vi "MAIN v1.vi"() -> ()   [LabVIEW 2012]
panel:
  out "REF-2 Block Check":i32
  in  "REF-2 Stream":bool
  out "REF-2":dbl[][](graph)
  in  "Bridge":string="PCB_REF"
  in  "Average Number":i32
  in  "Impact Location":i32
  out "Trailer":dbl[][](graph)
  in  "Trailer Stream":bool
  out "Trailer Block Check":i32
  out "error out":errorcluster
  out "REF Block Check":i32
  in  "REF-1 Stream":bool
  out "REF-1":dbl[][](graph)
  in  "Save Path:":path
  in  "?":bool
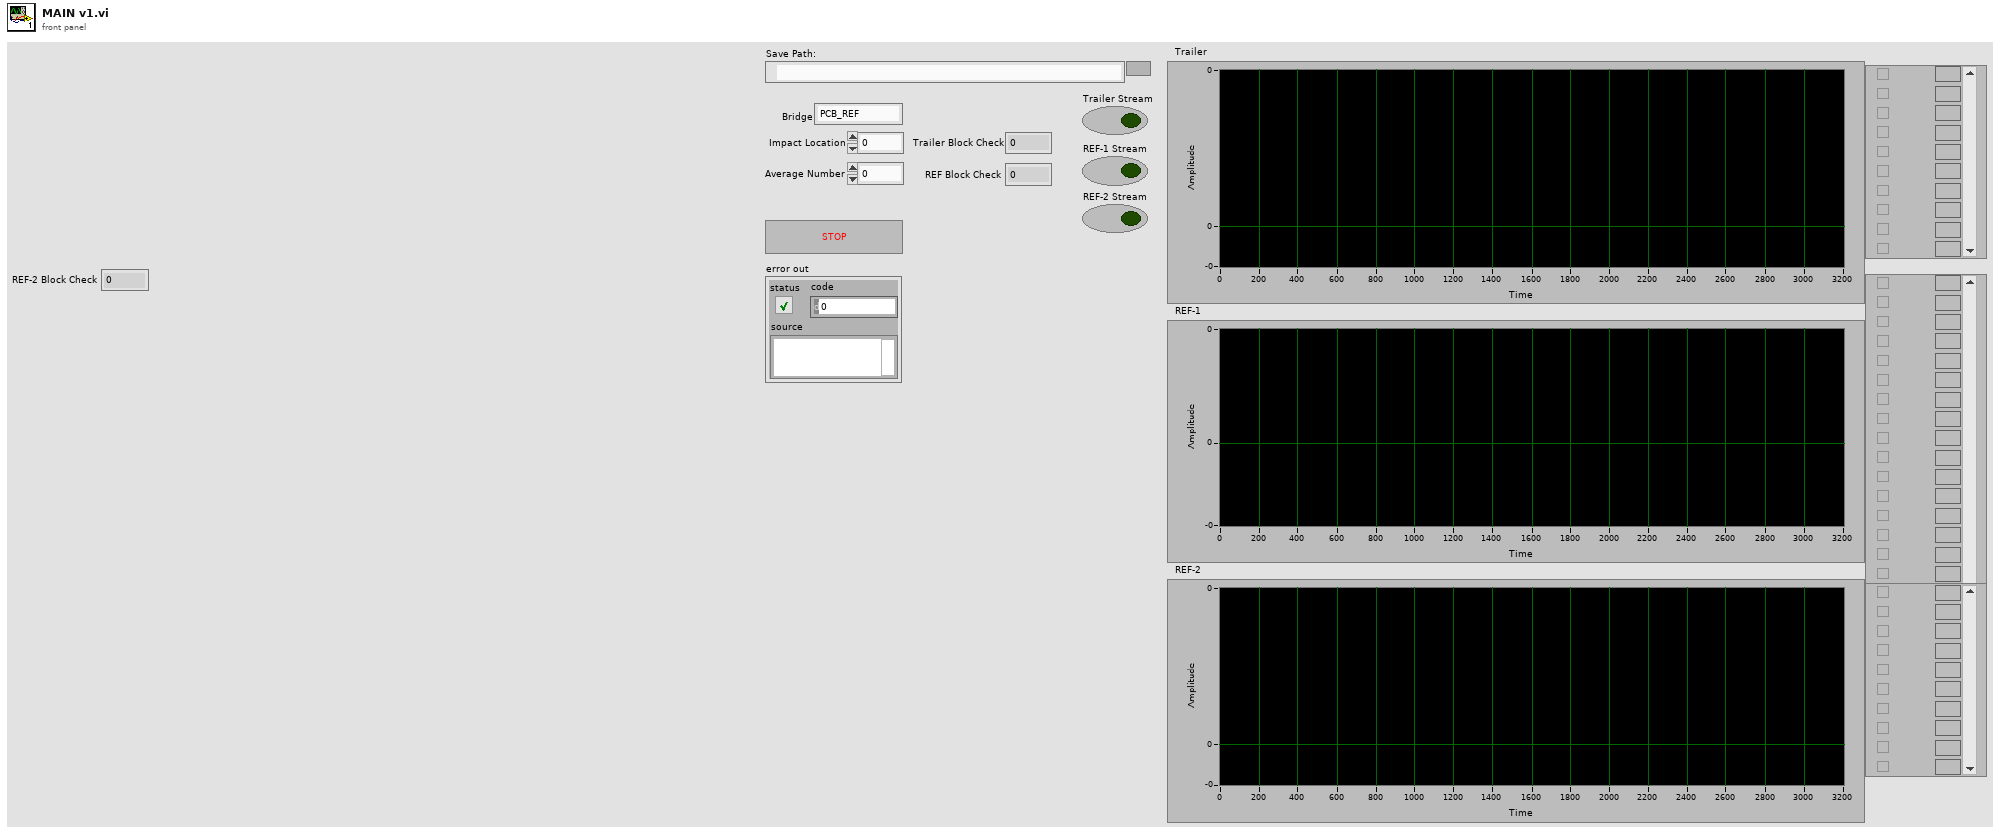
[diagram p1: front panel]
types:
  T1 = enum16{"open", "replace", "create", "open or create", "replace or create", "replace or create with confirmation"}
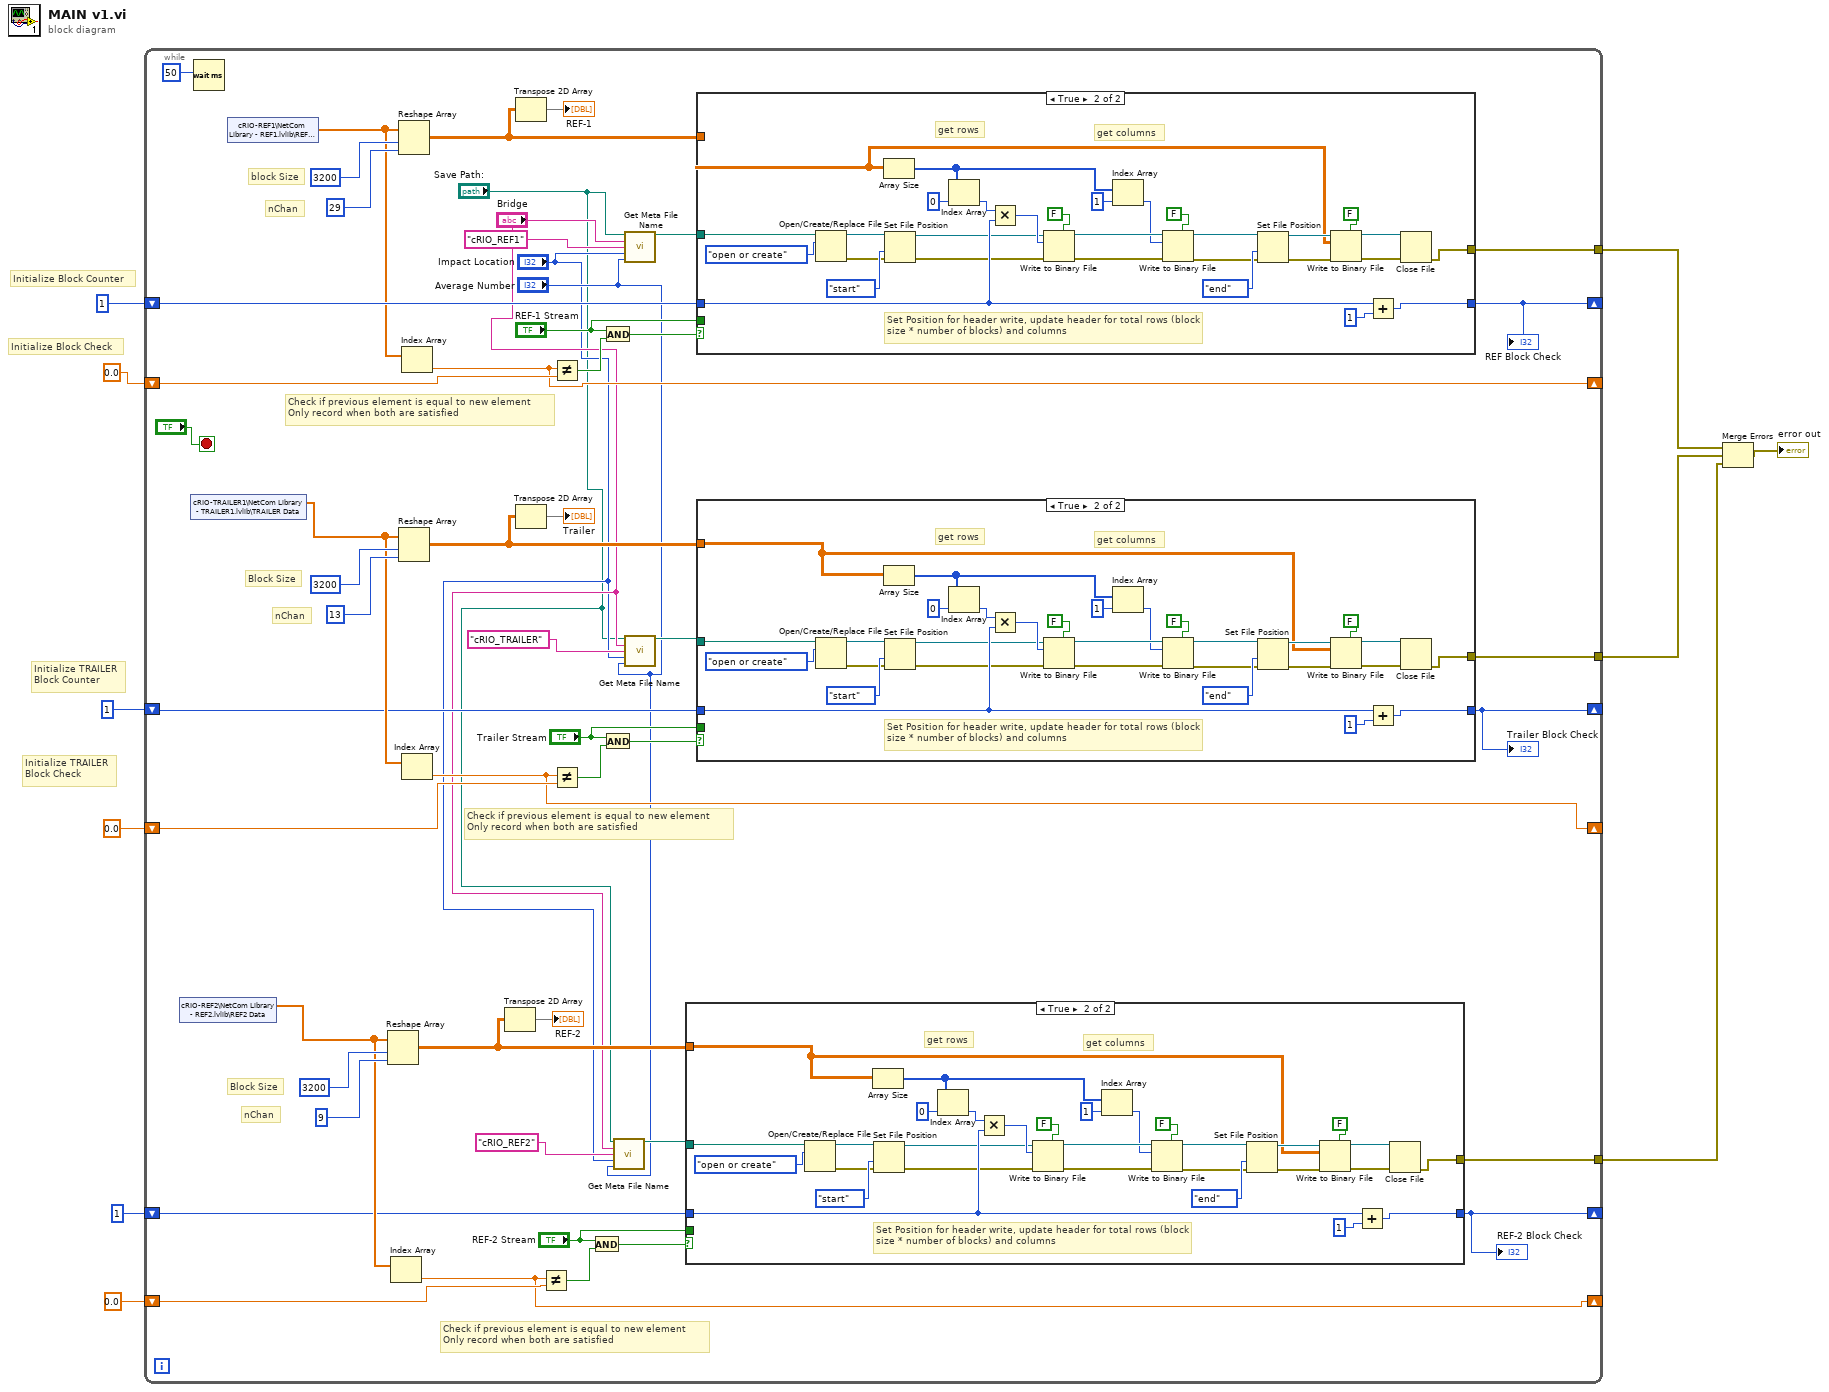
[diagram p0: block diagram]
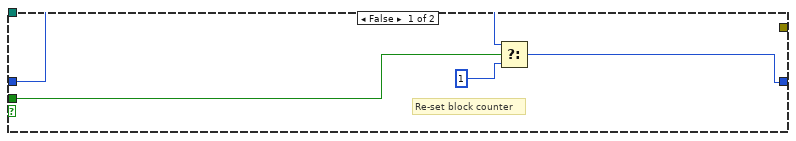
[diagram p2: hidden frame]
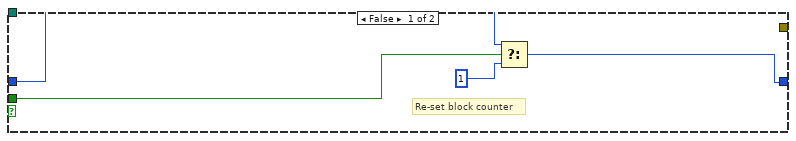
[diagram p3: hidden frame]
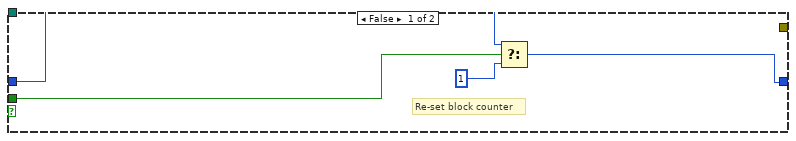
[diagram p4: hidden frame]
diagram:
  # "Initialize TRAILER\nBlock Check"
  # "Initialize TRAILER\nBlock Counter"
  # "Initialize Block Check"
  # "Initialize Block Counter"
  n1 = while {
    shift-right: [w56] -> _
    shift-left: 1 -> [w57]
    tunnel: [w52] -> w5
    shift-right: [w49] -> _
    shift-left: 0.0 -> [w50]
    shift-right: [w38] -> _
    shift-left: 1 -> [w37]
    shift-right: [w35] -> _
    shift-left: 0.0 -> [w36]
    tunnel: [w34] -> w6
    shift-right: [w14] -> _
    shift-left: 1 -> [w15]
    tunnel: [w13] -> w2
    shift-right: [w11] -> _
    shift-left: 0.0 -> [w12]
    stop <- "?" stop-if-true
    # "nChan"
    # "Block Size"
    # "nChan"
    # "Block Size"
    # "Check if previous element is equal to new element\nOnly record when both are satisfied"
    # "Check if previous element is equal to new element\nOnly record when both are satisfied"
    # "Check if previous element is equal to new element\nOnly record when both are satisfied"
    # "block Size"
    # "nChan"
    n2 = shared-variable "cRIO-REF2\\NetCom Library - REF2.lvlib\\REF2 Data"() -> (w22:dbl[])  [unwired: 1 in, 1 out]
    n3 = shared-variable "cRIO-TRAILER1\\NetCom Library - TRAILER1.lvlib\\TRAILER Data"() -> (w39:dbl[])  [unwired: 1 in, 1 out]
    n4 = Wait (ms)(milliseconds to wait=u32 50) -> ()  [unwired: 1 out]
    n5 = shared-variable "cRIO-REF1\\NetCom Library - REF1.lvlib\\REF Data"() -> (w51:dbl[])  [unwired: 1 in, 1 out]
    n6 = Reshape Array(w22, 3200, 9) -> (w23:dbl[][])
    n7 = Index Array(array=w22) -> (element=w11:dbl)  [unwired: 1 in]
    n8 = Reshape Array(w51, 3200, 29) -> (w59:dbl[][])
    n9 = Reshape Array(w39, 3200, 13) -> (w40:dbl[][])
    n10 = Index Array(array=w51) -> (element=w49:dbl)  [unwired: 1 in]
    n11 = Index Array(array=w39) -> (element=w35:dbl)  [unwired: 1 in]
    n12 = Transpose 2D Array(2D array=w23) -> (transposed array=→"REF-2":dbl[][])
    n13 = Transpose 2D Array(2D array=w59) -> (transposed array=→"REF-1":dbl[][])
    n14 = Transpose 2D Array(2D array=w40) -> (transposed array=→"Trailer":dbl[][])
    n15 = Not Equal?(x=w11, y=w12) -> (x != y?=w28:bool)
    n16 = Not Equal?(x=w49, y=w50) -> (x != y?=w48:bool)
    n17 = Not Equal?(x=w35, y=w36) -> (x != y?=w45:bool)
    n18 = And(x="REF-2 Stream", y=w28) -> (x .and. y?=w25:bool)
    n19 = And(x="REF-1 Stream", y=w48) -> (x .and. y?=w55:bool)
    n20 = And(x="Trailer Stream", y=w45) -> (x .and. y?=w42:bool)
    n21 = call "Get Meta File Name.vi"("Base Path"="Save Path:", "Bridge"="Bridge", "cRIO"="cRIO_REF2" ("Bridge/cRIO"), "Impact Location"="Impact Location", "Average Number"="Average Number") -> ("Full Path"=w21:path)  [unwired: 10 in]
    n22 = call "Get Meta File Name.vi"("Base Path"="Save Path:", "Bridge"="Bridge", "cRIO"="cRIO_REF1", "Impact Location"="Impact Location", "Average Number"="Average Number") -> ("Full Path"=w33:path)  [unwired: 10 in]
    n23 = call "Get Meta File Name.vi"("Base Path"="Save Path:", "Bridge"="Bridge", "cRIO"="cRIO_TRAILER" ("Bridge/cRIO"), "Impact Location"="Impact Location", "Average Number"="Average Number") -> ("Full Path"=w32:path)  [unwired: 10 in]
    n24 = case shown="True" w25 {
      tunnel: w23 -> [_ w68]
      tunnel: w15 -> [w64 w88]
      tunnel: [w63 w86] -> w14
      tunnel: w21 -> [_ w67]
      tunnel: [_ w66] -> w13
      tunnel: "REF-2 Stream" -> [w62 _]
      frame False {
        # "Re-set block counter"
        n25 = Select(t=w64, s=w62, f=1) -> (s? t:f=w63:i32)
      }
      frame True {
        # "get columns"
        # "Set Position for header write, update header for total rows (block size * number of blocks) and columns"
        # "get rows"
        n26 = Open/Create/Replace File(file path (use dialog)=w67, operation (0:open)=T1."open or create") -> (refnum out=w93:refnum<file>, error out=w91:errorcluster)  [unwired: 4 in, 1 out]
        n27 = Array Size(array=w68) -> (size(s)=w81:i32[])
        n28 = Set File Position(refnum=w93, from (0:start)=enum16{"start", "end", "current"}."start", error in=w91) -> (refnum out=w84:refnum<file>, error out=w83:errorcluster)  [unwired: 1 in]
        n29 = Index Array(array=w81, index=0) -> (element=w89:i32)
        n30 = Multiply(x=w89, y=w88) -> (x*y=w85:i32)
        n31 = Write to Binary File(file (use dialog)=w84, data=w85, error in=w83, 5:FALSE ("prepend array or string size? (T)")) -> (refnum out=w79:refnum<file>, error out=w78:errorcluster)  [unwired: 2 in, 1 out]
        n32 = Index Array(array=w81, index=1) -> (element=w77:i32)
        n33 = Write to Binary File(file (use dialog)=w79, data=w77, error in=w78, 5:FALSE ("prepend array or string size? (T)")) -> (refnum out=w74:refnum<file>, error out=w75:errorcluster)  [unwired: 2 in, 1 out]
        n34 = Set File Position(refnum=w74, from (0:start)=enum16{"start", "end", "current"}."end", error in=w75) -> (refnum out=w72:refnum<file>, error out=w73:errorcluster)  [unwired: 1 in]
        n35 = Write to Binary File(file (use dialog)=w72, data=w68, error in=w73, 5:FALSE ("prepend array or string size? (T)")) -> (refnum out=w69:refnum<file>, error out=w70:errorcluster)  [unwired: 2 in, 1 out]
        n36 = Add(x=w88, y=1) -> (x+y=w86:i32)
        n37 = Close File(refnum=w69, error in=w70) -> (error out=w66:errorcluster)  [unwired: 1 out]
      }
    }
    "REF-2 Block Check" <- w14
    n38 = case shown="True" w55 {
      tunnel: w59 -> [_ w136]
      tunnel: w57 -> [w132 w156]
      tunnel: [w131 w154] -> w56
      tunnel: w33 -> [_ w135]
      tunnel: [_ w134] -> w52
      tunnel: "REF-1 Stream" -> [w130 _]
      frame False {
        # "Re-set block counter"
        n39 = Select(t=w132, s=w130, f=1) -> (s? t:f=w131:i32)
      }
      frame True {
        # "get columns"
        # "Set Position for header write, update header for total rows (block size * number of blocks) and columns"
        # "get rows"
        n40 = Open/Create/Replace File(file path (use dialog)=w135, operation (0:open)=T1."open or create") -> (refnum out=w161:refnum<file>, error out=w159:errorcluster)  [unwired: 4 in, 1 out]
        n41 = Array Size(array=w136) -> (size(s)=w149:i32[])
        n42 = Set File Position(refnum=w161, from (0:start)=enum16{"start", "end", "current"}."start", error in=w159) -> (refnum out=w152:refnum<file>, error out=w151:errorcluster)  [unwired: 1 in]
        n43 = Index Array(array=w149, index=0) -> (element=w157:i32)
        n44 = Multiply(x=w157, y=w156) -> (x*y=w153:i32)
        n45 = Write to Binary File(file (use dialog)=w152, data=w153, error in=w151, 5:FALSE ("prepend array or string size? (T)")) -> (refnum out=w147:refnum<file>, error out=w146:errorcluster)  [unwired: 2 in, 1 out]
        n46 = Index Array(array=w149, index=1) -> (element=w145:i32)
        n47 = Write to Binary File(file (use dialog)=w147, data=w145, error in=w146, 5:FALSE ("prepend array or string size? (T)")) -> (refnum out=w142:refnum<file>, error out=w143:errorcluster)  [unwired: 2 in, 1 out]
        n48 = Set File Position(refnum=w142, from (0:start)=enum16{"start", "end", "current"}."end", error in=w143) -> (refnum out=w140:refnum<file>, error out=w141:errorcluster)  [unwired: 1 in]
        n49 = Write to Binary File(file (use dialog)=w140, data=w136, error in=w141, 5:FALSE ("prepend array or string size? (T)")) -> (refnum out=w137:refnum<file>, error out=w138:errorcluster)  [unwired: 2 in, 1 out]
        n50 = Add(x=w156, y=1) -> (x+y=w154:i32)
        n51 = Close File(refnum=w137, error in=w138) -> (error out=w134:errorcluster)  [unwired: 1 out]
      }
    }
    "REF Block Check" <- w56
    n52 = case shown="True" w42 {
      tunnel: w40 -> [_ w102]
      tunnel: w37 -> [w98 w122]
      tunnel: [w97 w120] -> w38
      tunnel: w32 -> [_ w101]
      tunnel: [_ w100] -> w34
      tunnel: "Trailer Stream" -> [w96 _]
      frame False {
        # "Re-set block counter"
        n53 = Select(t=w98, s=w96, f=1) -> (s? t:f=w97:i32)
      }
      frame True {
        # "get columns"
        # "Set Position for header write, update header for total rows (block size * number of blocks) and columns"
        # "get rows"
        n54 = Open/Create/Replace File(file path (use dialog)=w101, operation (0:open)=T1."open or create") -> (refnum out=w127:refnum<file>, error out=w125:errorcluster)  [unwired: 4 in, 1 out]
        n55 = Array Size(array=w102) -> (size(s)=w115:i32[])
        n56 = Set File Position(refnum=w127, from (0:start)=enum16{"start", "end", "current"}."start", error in=w125) -> (refnum out=w118:refnum<file>, error out=w117:errorcluster)  [unwired: 1 in]
        n57 = Index Array(array=w115, index=0) -> (element=w123:i32)
        n58 = Multiply(x=w123, y=w122) -> (x*y=w119:i32)
        n59 = Write to Binary File(file (use dialog)=w118, data=w119, error in=w117, 5:FALSE ("prepend array or string size? (T)")) -> (refnum out=w113:refnum<file>, error out=w112:errorcluster)  [unwired: 2 in, 1 out]
        n60 = Index Array(array=w115, index=1) -> (element=w111:i32)
        n61 = Write to Binary File(file (use dialog)=w113, data=w111, error in=w112, 5:FALSE ("prepend array or string size? (T)")) -> (refnum out=w108:refnum<file>, error out=w109:errorcluster)  [unwired: 2 in, 1 out]
        n62 = Set File Position(refnum=w108, from (0:start)=enum16{"start", "end", "current"}."end", error in=w109) -> (refnum out=w106:refnum<file>, error out=w107:errorcluster)  [unwired: 1 in]
        n63 = Write to Binary File(file (use dialog)=w106, data=w102, error in=w107, 5:FALSE ("prepend array or string size? (T)")) -> (refnum out=w103:refnum<file>, error out=w104:errorcluster)  [unwired: 2 in, 1 out]
        n64 = Add(x=w122, y=1) -> (x+y=w120:i32)
        n65 = Close File(refnum=w103, error in=w104) -> (error out=w100:errorcluster)  [unwired: 1 out]
      }
    }
    "Trailer Block Check" <- w38
  }
  n66 = Merge Errors(w5, w6, w2) -> (→"error out":errorcluster)
